vi "Read ADC.vi"(8 "error in (no error)":errorcluster, 9 "Canal":u8, 10 "VISA resource name":refnum<visa-resource-name>, 11 "Arduino in":refnum<class "Arduino.lvclass">) -> (0 "error out":errorcluster, 1 "Response":i32, 2 "VISA resource name 2":refnum<visa-resource-name>, 3 "Arduino out":refnum<class "Arduino.lvclass">)   [LabVIEW 2020, in "Arduino.lvclass"]
uses:
  Arduino.lvclass
  42acfc40-328b-4b97-b9ff-c8cea09297f2.vi
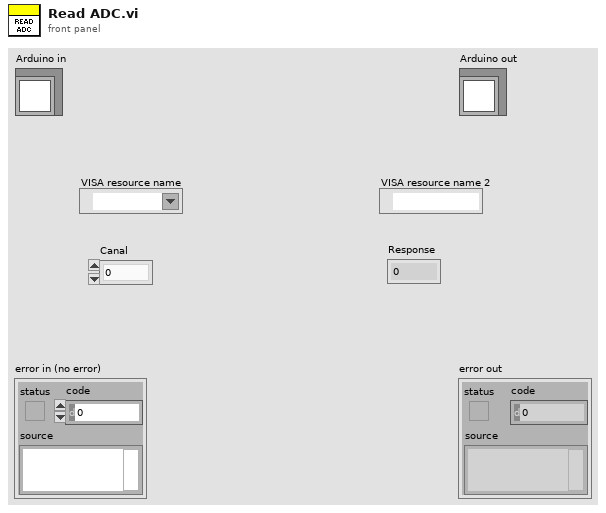
[diagram p1: front panel]
types:
  T1 = enum16{"Write", "Read", "Config", "Reset", "Close"}
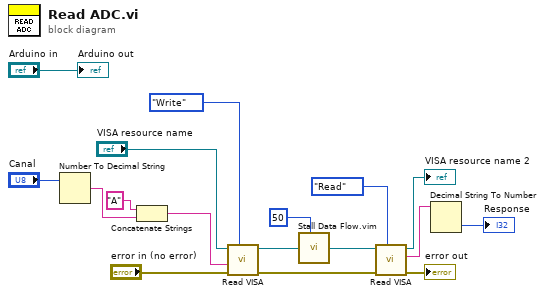
[diagram p0: block diagram]
diagram:
  n1 = Number To Decimal String(number="Canal") -> (decimal integer string=w12:string)  [unwired: 1 in]
  n2 = Concatenate Strings("A" ("string"), w12) -> (w11:string)
  n3 = call "Read VISA.vi"("Opciones"=T1."Write", "error in (no error)"="error in (no error)", "Write"=w11, "VISA com port"="VISA resource name") -> ("error out"=w6:errorcluster, "VISA com port 2"=w9:refnum<visa-resource-name>)  [unwired: 5 in, 1 out]
  n4 = call "Stall Data Flow.vim"("value in"=w9, "milliseconds to wait"=u32 50) -> ("value out"=w8:refnum<visa-resource-name>)  [unwired: 1 out]
  n5 = call "Read VISA.vi"("Opciones"=T1."Read", "error in (no error)"=w6, "VISA com port"=w8) -> ("error out"=→"error out":errorcluster, "Read"=w3:string, "VISA com port 2"=→"VISA resource name 2":refnum<visa-resource-name>)  [unwired: 6 in]
  n6 = Decimal String To Number(string=w3) -> (number=→"Response":i32)  [unwired: 2 in, 1 out]
  "Arduino out" <- "Arduino in"
